vi "SubVI_Apenas_Ang_Positivo.vi"(1 "Ang_entrada":dbl) -> (0 "Ang_saida":dbl)   [LabVIEW 2017]
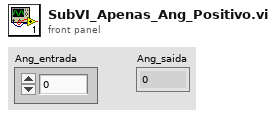
[diagram p1: front panel]
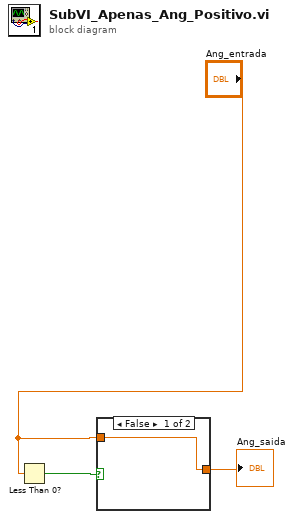
[diagram p0: block diagram]
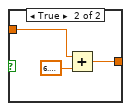
[diagram p2: hidden frame]
diagram:
  n1 = Less Than 0?(x="Ang_entrada") -> (x < 0?=w1:bool)
  n2 = case shown="False" w1 {
    tunnel: "Ang_entrada" -> [w4 w7]
    tunnel: [w4 w5] -> w3
    frame False {
    }
    frame True {
      n3 = Add(x=w7, y=6.283185307179586) -> (x+y=w5:dbl)
    }
  }
  "Ang_saida" <- w3
